vi "Main Comm Loops.vi"(6 "Update Rate":u32=10, 8 "error in (no error)":errorcluster, 10 "Comm.lvclass":refnum<class "VeriStand Comm.lvclass">, 11 "Process":refnum<class "Process.lvclass">) -> (0 "error out":errorcluster)   [LabVIEW 2019, in "NI VeriStand Addon Network Comm.lvlib" / "VeriStand Comm.lvclass"]
uses:
  VeriStand Comm.lvclass
  <vilib>/NI/NIVS Inline Async API/_VS Inline Async API/Process/Process.lvclass
  VeriStand Comm.lvclass/VeriStand Comm.ctl
  <vilib>/NI/NIVS Inline Async API/_VS Inline Async API/Process/Process.lvclass/Process.ctl
  <vilib>/NI/STM/Connection Manager/TCP/Advanced/TCP Connection Manager (By Reference).vi
  <vilib>/Utility/error.llb/Clear Errors.vi
  <vilib>/NI/STM/Get Connection Reference.vi
  <vilib>/NI/STM/TCP/Get Connection Reference (TCP).vi
  <vilib>/NI/STM/Read Meta Data.vi
  <vilib>/NI/STM/TCP/Read Meta Data (TCP Ref).vi
  <vilib>/NI/NIVS Inline Async API/_VS Inline Async API/Process/Methods/Async.Processes.Report.vi
  <vilib>/NI/AMC/Send Local Message.vi
  <vilib>/NI/Tools/Keyed Array/Add.vi
  <vilib>/NI/AMC/Read Next Message.vi
  <vilib>/NI/STM/Connection Manager/TCP/Advanced/TCP Check Connection (By Reference).vi
  <vilib>/NI/STM/SubVIs/Generate STM Error.vi
  <vilib>/NI/NIVS Inline Async API/_VS Inline Async API/Error Handling Process/SubVIs/Error.ConvertArray.vi
  <vilib>/NI/AMC/Create Single Message.vi
  <vilib>/NI/AMC/Update Message Routing Info.vi
  <vilib>/NI/Tools/Keyed Array/Map String.vi
  <vilib>/NI/AMC/Read Termination Message.vi
  <vilib>/NI/Tools/String/Get Case Matching.vi
  <vilib>/NI/STM/Read Message.vi
  <vilib>/NI/STM/TCP/Read Message (TCP).vi
  <vilib>/NI/AMC/Send Message.vi
  Shared/Comm Constants.vi
  <vilib>/NI/AMC/Create Message Queue.vi
  <vilib>/NI/AMC/Globals.vi
  <vilib>/NI/STM/Write Message.vi
  <vilib>/NI/STM/TCP/Write Message (TCP).vi
  <vilib>/NI/AMC/Destroy Message Queue.vi
  <vilib>/Utility/SystemLogging/Write to System Log.vi
  <vilib>/NI/STM/TCP/Read Meta Data (TCP Clst).vi
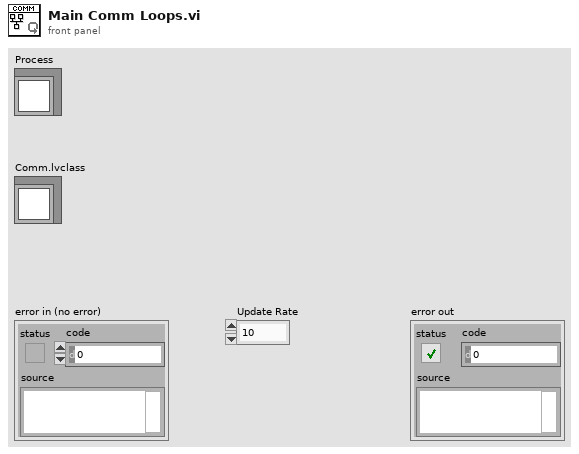
[diagram p1: front panel]
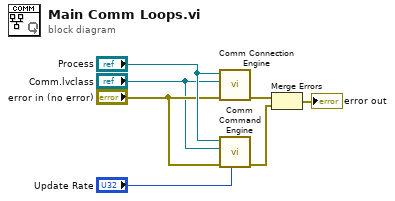
[diagram p0: block diagram]
diagram:
  n1 = call "Comm Connection Engine.vi"("error in (no error)"="error in (no error)", "Comm.lvclass"="Comm.lvclass", "Process"="Process") -> ("error out"=w4:errorcluster)  [unwired: 8 in]
  n2 = call "Comm Command Engine.vi"("Loop Time (ms)"="Update Rate", "error in (no error)"="error in (no error)", "Comm.lvclass"="Comm.lvclass", "Process"="Process") -> ("error out"=w3:errorcluster)  [unwired: 7 in]
  n3 = Merge Errors(w4, w3) -> (→"error out":errorcluster)
